vi "hse-application_DetermineFrameworkVersionNumber.vi"(8 "error in":errorcluster, 11 "Application in":refnum<class "hse-application.lvclass">) -> (0 "error out":errorcluster, 3 "Application out":refnum<class "hse-application.lvclass">)   [LabVIEW 2022 SP3, in "hse-application.lvclass"]
doc: "Sets the version of the framework used for the application.\n\n____\nHAMPEL SOFTWARE ENGINEERING v3.8.0 (2023-12-18 14:41)"
uses:
  hse-application.lvclass
  hse-application.lvclass/hse-application.ctl
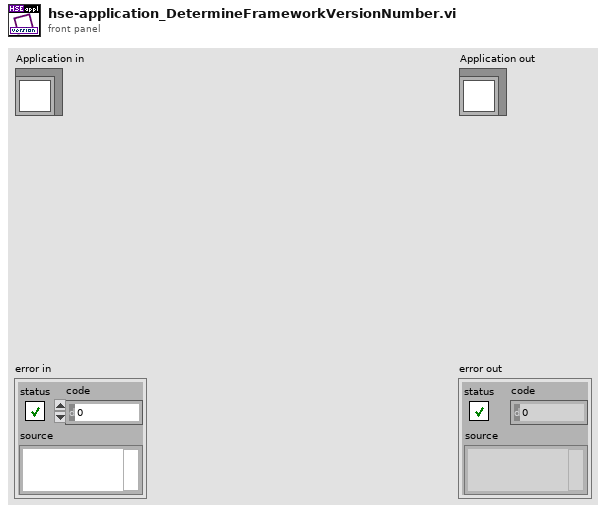
[diagram p1: front panel]
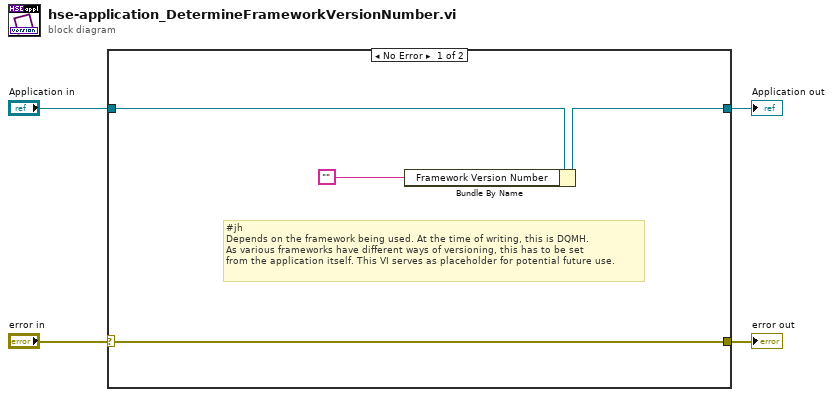
[diagram p0: block diagram]
diagram:
  n1 = case shown="No Error" "error in" {
    selector: "error in" -> [w6 w10]
    tunnel: [w6 w10] -> w3
    tunnel: [w7 w9] -> w1
    tunnel: "Application in" -> [w8 w9]
    frame No Error {
      # "#jh \nDepends on the framework being used. At the time of writing, this is DQMH.\nAs various frameworks have different ways of versioning, this has to be set\nfrom the application itself. This VI serves as placeholder for potential future use."
      n2 = Bundle By Name(cluster=w8, "Framework Version Number"="") -> (w7:refnum<class "hse-application.lvclass">)
    }
    frame Error {
    }
  }
  "error out" <- w3
  "Application out" <- w1
